vi "output.vi"(8 "error in":errorcluster, 10 "data table in":T1, 11 "bin datalogger runtime in":refnum<class "Binary datalogger runtime.lvclass">) -> (0 "error out":errorcluster, 2 "data table out":T1, 3 "bin datalogger runtime out":refnum<class "Binary datalogger runtime.lvclass">)   [LabVIEW 2013, in "Binary datalogger runtime.lvclass"]
doc: "Provides an interface for writing data to a module at runtime. While this interface performs no operations, a child should provide an override which may write to any open sessions, references, or interfaces."
uses:
  Binary datalogger runtime.lvclass
  <vilib>/NI/Tag Bus/table/data table.ctl
  Binary datalogger runtime.lvclass/Binary datalogger runtime.ctl
  response from background process.ctl
  response enum.ctl
  message to background process.ctl
  control enum.ctl
  <vilib>/NI/Tag Bus/table/data table.lvlib
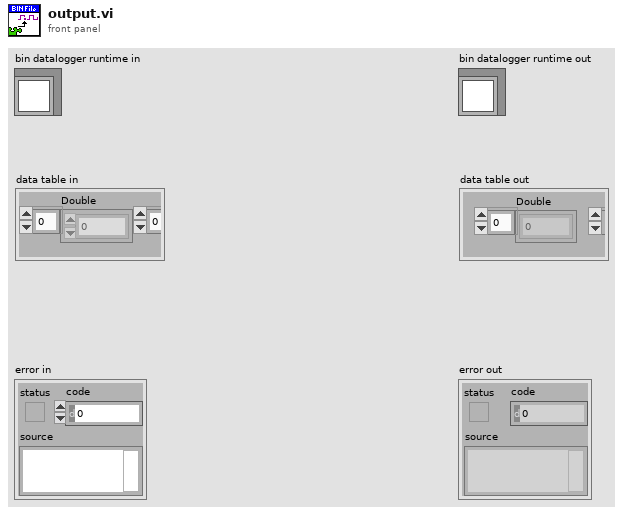
[diagram p1: front panel]
types:
  T1 = typedef "tag bus.lvlib/data table.lvlib/data table.ctl" = cluster{"Double":dbl[], "Single":sgl[], "I64":i64[], "I32":i32[], "I16":i16[], "I8":i8[], "U64":u64[], "U32":u32[], "U16":u16[], "U8":u8[], "Boolean":bool[], "String":string[], "Array of Double":cluster{"DBL Array":dbl[]}[], "Array of Single":cluster{"SGL Array":sgl[]}[], "Array of I64":cluster{"I64 Array":i64[]}[], "Array of I32":cluster{"I32 Array":i32[]}[], "Array of I16":cluster{"I16 Array":i16[]}[], "Array of I8":cluster{"I8 Array":i8[]}[], "Array of U64":cluster{"U64 Array":u64[]}[], "Array of U32":cluster{"U32 Array":u32[]}[], "Array of U16":cluster{"U16 Array":u16[]}[], "Array of U8":cluster{"U8 Array":u8[]}[], "Array of Boolean":cluster{"Boolean Array":bool[]}[], "Array of String":cluster{"String Array":string[]}[]}
  T2 = typedef "Binary datalogger runtime.lvclass/response from background process.ctl" = cluster{"response enum":T3, "datapack":refnum<data-value>, "error code":i32}
  T3 = typedef "Binary datalogger runtime.lvclass/response enum.ctl" = enum16{"exit", "return buffer", "error"}
  T4 = typedef "TDMS datalogger runtime.lvclass/response from background process.ctl" = cluster{"response enum":T5, "datapack":refnum<data-value>, "error code":i32}
  T5 = typedef "TDMS datalogger runtime.lvclass/response enum.ctl" = enum16{"exit", "return buffer", "error"}
  T6 = typedef "Binary datalogger runtime.lvclass/control enum.ctl" = enum16{"exit", "output data"}
  T7 = typedef "Binary datalogger runtime.lvclass/message to background process.ctl" = cluster{"control enum":T6, "datapack":refnum<data-value>, "Time Stamp":timestamp}
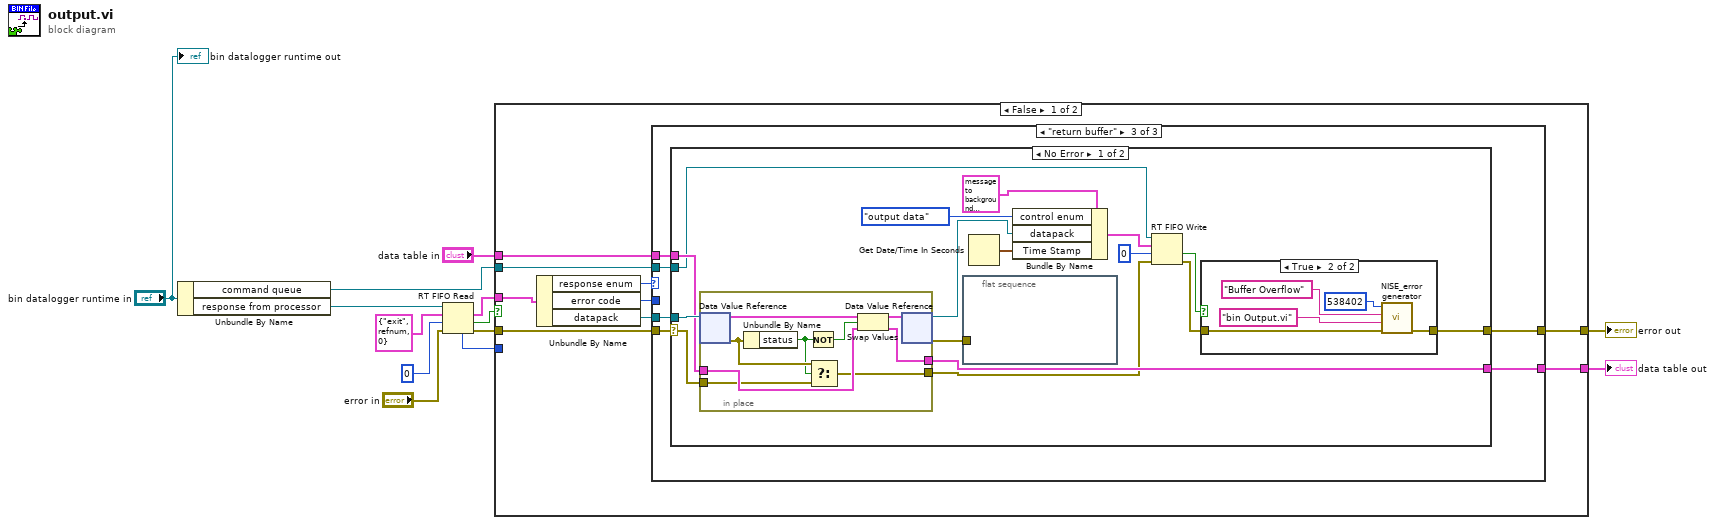
[diagram p0: block diagram]
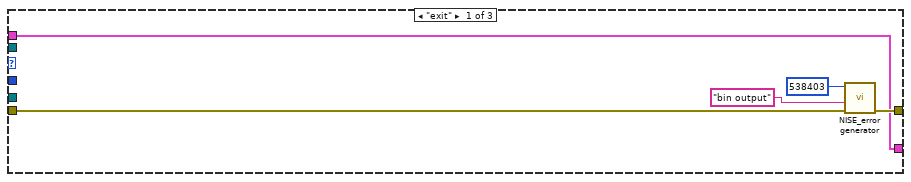
[diagram p2: hidden frame]
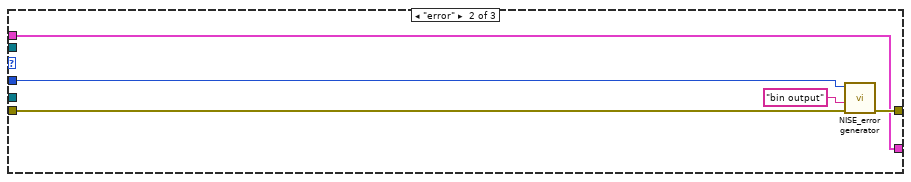
[diagram p3: hidden frame]
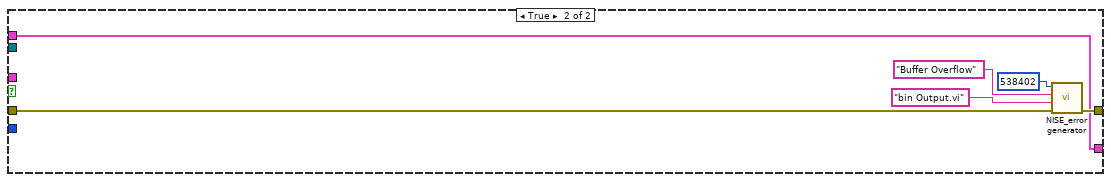
[diagram p6: hidden frame]
diagram:
  n1 = Unbundle By Name("bin datalogger runtime in") -> ("command queue"=w3:refnum<k33>, "response from processor"=w12:refnum<k33>)
  n2 = RT FIFO Read(0:w12, 1:T2 {"response enum"=enum."exit", "datapack"=refnum, "error code"=0} ("element"), 2:0 ("timeout in ms (0)"), 3:"error in") -> (7:w4:u32, 9:w9:T4, 10:w10:bool, 11:w8:errorcluster)  [unwired: 1 out]
  n3 = case shown="False" w10 {
    tunnel: w9 -> [w22 _]
    tunnel: w8 -> [w19 w77]
    tunnel: [w20 w76] -> w5
    tunnel: w4 -> [_ _]
    tunnel: w3 -> [w16 _]
    tunnel: "data table in" -> [w15 w72]
    tunnel: [w14 w72] -> w1
    frame False {
      n4 = Unbundle By Name(w22) -> ("response enum"=w21:T5, "error code"=w18:i32, "datapack"=w17:refnum<data-value>)
      n5 = case shown="\"return buffer\"" w21 {
        tunnel: [w26 w31 w35] -> w20
        tunnel: w19 -> [w27 w32 w36]
        tunnel: w18 -> [_ w30 _]
        tunnel: w17 -> [_ _ w38]
        tunnel: w16 -> [_ _ w37]
        tunnel: w15 -> [w23 w28 w34]
        tunnel: [w23 w28 w33] -> w14
        frame "exit" {
          n6 = call <vilib>:"NISE_error generator.vi"("error in"=w27, "source"="bin output", "error code (0)"=538403) -> ("error out"=w26:errorcluster)  [unwired: 6 in]
        }
        frame "error" {
          n7 = call <vilib>:"NISE_error generator.vi"("error in"=w32, "source"="bin output", "error code (0)"=w30) -> ("error out"=w31:errorcluster)  [unwired: 6 in]
        }
        frame "return buffer" {
          n8 = case shown="No Error" w36 {
            selector: w36 -> [w50 w71]
            tunnel: w38 -> [w54 _]
            tunnel: w37 -> [w48 _]
            tunnel: [w39 w71] -> w35
            tunnel: w34 -> [w53 w70]
            tunnel: [w52 w70] -> w33
            frame No Error {
              n9 = in-place {
                in-place-border: w53 -> [w69]
                in-place-border: [w67] -> w52
                in-place-border: w50 -> [w63]
                in-place-border: [w61] -> w49
                n10 = in-place-dvr #1(w54) -> (w65:T1, w64:errorcluster)
                n11 = Unbundle By Name(w64) -> ("status"=w62:bool)
                n12 = Not(x=w62) -> (.not. x?=w68:bool)
                n13 = Select(t=w64, s=w62, f=w63) -> (s? t:f=w61:errorcluster)
                n14 = Swap Values(12:w65, 13:w68, 14:w69) -> (1:w66:T1, 3:w67:T1)
                n15 = in-place-dvr #1(w66) -> (w44:refnum<data-value>, w51:errorcluster)
              }
              n16 = flat-sequence {
                tunnel: w51 -> [_]
                frame #0 {
                }
              }
              n17 = Get Date/Time In Seconds() -> (seconds since 1Jan1904=w45:timestamp)
              n18 = Bundle By Name(cluster=T7 {"control enum"=enum."exit", "datapack"=refnum, "Time Stamp"=timestamp(0 s since 1904-01-01)} ("element"), "control enum"=control_enum."output data", "datapack"=w44, "Time Stamp"=w45) -> (w46:T7)
              n19 = RT FIFO Write(0:w48, 1:w46, 2:0 ("timeout in ms (0)"), 3:w49) -> (10:w41:bool, 11:w40:errorcluster)  [unwired: 1 in, 2 out]
              n20 = case shown="True" w41 {
                tunnel: w40 -> [w55 w57]
                tunnel: [w55 w56] -> w39
                frame False {
                }
                frame True {
                  n21 = call <vilib>:"NISE_error generator.vi"("error in"=w57, "source"="bin Output.vi", "append error message"="Buffer Overflow", "error code (0)"=538402 ("code")) -> ("error out"=w56:errorcluster)  [unwired: 5 in]
                }
              }
            }
            frame Error {
            }
          }
        }
      }
    }
    frame True {
      n22 = call <vilib>:"NISE_error generator.vi"("error in"=w77, "source"="bin Output.vi", "append error message"="Buffer Overflow", "error code (0)"=538402 ("code")) -> ("error out"=w76:errorcluster)  [unwired: 5 in]
    }
  }
  "error out" <- w5
  "data table out" <- w1
  "bin datalogger runtime out" <- "bin datalogger runtime in"
